vi "Rcv Cmd.vi"(8 "error in":errorcluster, 11 "nPAS in":refnum<class "nPAS.lvclass">) -> (0 "error out":errorcluster, 3 "nPAS out":refnum<class "nPAS.lvclass">)   [LabVIEW 2018, in "gPAS Library.lvlib" / "nPAS.lvclass"]
doc: "The override of the <b>Instrument:Rcv Cmd</b> method accounts for checking for speaker switching when the object is set to autocycle. How the change in switch state is executed is left to the <b>Change Speaker State</b> command object which is sent when the state is to be changed."
uses:
  nPAS.lvclass
  C:/Program Files (x86)/National Instruments/LabVIEW 2018/vi.lib/MSR Consulting, LLC/General Reuse/PAS/Main/PAS.lvclass
  C:/Program Files (x86)/National Instruments/LabVIEW 2018/vi.lib/MSR Consulting, LLC/General Reuse/Instrument/Instrument.lvclass
  <vilib>/MSR Consulting, LLC/General Reuse/PAS/Data/Main/PAS Data.lvclass
  <vilib>/MSR Consulting, LLC/General Reuse/Instrument/Instrument.lvclass/Instrument.ctl
  <vilib>/MSR Consulting, LLC/General Reuse/PAS/Cell/PAS Cell.lvclass/PAS Cell.ctl
  Commands/Change Laser Frequency Cmd/Change Laser Frequency CMD.lvclass
  C:/Program Files (x86)/National Instruments/LabVIEW 2018/vi.lib/MSR Consulting, LLC/General Reuse/Command/Command.lvclass
  Commands/Change Laser Frequency Cmd/Change Laser Frequency CMD.lvclass/Change Laser Frequency CMD.ctl
  Commands/Change Laser Frequency Cmd/Write Cell.vi
  Commands/Change Laser Frequency Cmd/Write f.vi
  <vilib>/MSR Consulting, LLC/General Reuse/PAS/Cell/Read speaker.vi
  <vilib>/MSR Consulting, LLC/General Reuse/Instrument/Read Data.vi
  <vilib>/MSR Consulting, LLC/General Reuse/Instrument/Read CMD.vi
  <vilib>/MSR Consulting, LLC/General Reuse/PAS/Main/Read Cells.vi
  <vilib>/MSR Consulting, LLC/General Reuse/PAS/Data/Main/Read CellData.vi
  <vilib>/MSR Consulting, LLC/General Reuse/PAS/Data/Cell/Read f0.vi
  <vilib>/MSR Consulting, LLC/General Reuse/PAS/Cell/PAS Cell.lvclass
  <vilib>/MSR Consulting, LLC/General Reuse/Data/Data.lvclass
  <vilib>/MSR Consulting, LLC/General Reuse/Command/Command.lvclass
  <vilib>/MSR Consulting, LLC/General Reuse/PAS/Data/Cell/PAS Cell Data.lvclass
  <vilib>/MSR Consulting, LLC/General Reuse/PAS/Main/PAS.lvclass
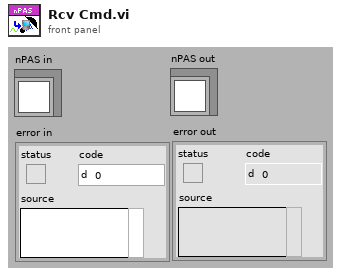
[diagram p1: front panel]
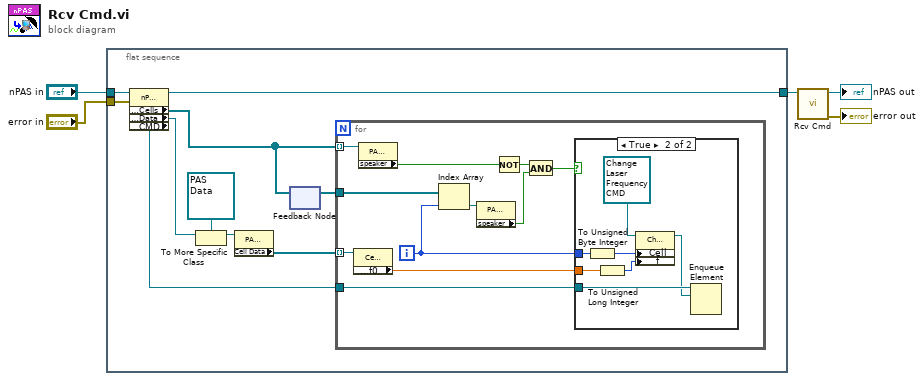
[diagram p0: block diagram]
diagram:
  n1 = flat-sequence {
    tunnel: "nPAS in" -> [w15]
    tunnel: "error in" -> [w14]
    tunnel: [w13] -> w2
    frame #0 {
      n2 = property class="nPAS"(reference=w15, error in=w14) -> (reference out=w13:refnum<class "nPAS.lvclass">, "Data Access:Cells"=w7:refnum<class "PAS Cell.lvclass">[], "Accessors:Data"=w12:refnum<class "Data.lvclass">, "Accessors:CMD"=w8:refnum<queue>)  [unwired: 1 out]
      n3 = To More Specific Class(target class=refnum<class "PAS Data.lvclass"> refnum ("PAS Library.lvlib:PAS Data"), reference=w12) -> (specific class reference=w10:refnum<class "PAS Data.lvclass">)  [unwired: 1 in, 1 out]
      n4 = property class="PAS Data"(reference=w10) -> ("Cell Data"=w9:refnum<class "PAS Cell Data.lvclass">[])  [unwired: 1 in, 2 out]
      n5 = feedback #1() -> (w6:refnum<class "PAS Cell.lvclass">[])  [unwired: 1 in]
      n6 = feedback-in #1(w7) -> ()
      n7 = for {
        tunnel: w7 -> [w26] mode=indexing
        tunnel: w9 -> [w22] mode=indexing
        tunnel: w8 -> [w21]
        tunnel: w6 -> [w19]
        i -> [w18]
        n8 = property class="Cell Data"(reference=w22) -> ("Accessors:f0"=w20:sgl)  [unwired: 1 in, 2 out]
        n9 = property class="PAS Cell"(reference=w26) -> ("speaker"=w25:bool)  [unwired: 1 in, 2 out]
        n10 = Index Array(array=w19, index=w18) -> (element=w17:refnum<class "PAS Cell.lvclass">)
        n11 = property class="PAS Cell"(reference=w17) -> ("speaker"=w16:bool)  [unwired: 1 in, 2 out]
        n12 = Not(x=w25) -> (.not. x?=w24:bool)
        n13 = And(x=w24, y=w16) -> (x .and. y?=w23:bool)
        n14 = case shown="True" w23 {
          tunnel: w21 -> [_ w28]
          tunnel: w20 -> [_ w32]
          tunnel: w18 -> [_ w30]
          frame False {
          }
          frame True {
            n15 = To Unsigned Byte Integer(number=w30) -> (unsigned 8bit integer=w29:u8)
            n16 = To Unsigned Long Integer(number=w32) -> (unsigned 32bit integer=w31:u32)
            n17 = property class="Change Laser Frequency CMD"(reference=refnum<class "Change Laser Frequency CMD.lvclass"> refnum ("gPAS Library.lvlib:Change Laser Frequency CMD"), "Cell"=w29, "f"=w31) -> (reference out=w27:refnum<class "Change Laser Frequency CMD.lvclass">)  [unwired: 1 in, 1 out]
            n18 = Enqueue Element(queue=w28, element=w27) -> ()  [unwired: 2 in, 3 out]
          }
        }
      }
    }
  }
  n19 = call-parent "Rcv Cmd.vi"("PAS in"=w2) -> ("error out"=→"error out":errorcluster, "PAS out"=→"nPAS out":refnum<class "nPAS.lvclass">)  [unwired: 9 in]
